vi "LabVIEW_Switch_State_Detection.vi"() -> ()   [LabVIEW 2020]
uses:
  <vilib>/Instr/_visa.llb/Select Event Type.ctl
  <vilib>/Instr/_visa.llb/VISA Configure Serial Port (Instr).vi
panel:
  in  "Stop":bool
  in  "Tab Control":T1(tab)
  out "Switch 1":bool
  out "Serial Read Buffer":string
  in  "VISA resource name":refnum<visa-resource-name>="COM17"
  in  "baud rate (9600)":u32=9600
  out "Reading Rate (ms)":u32
  out "Switch 2":bool
  # "Switch State Detection with Arduino and LabVIEW"
  # "Auther: Suparat Yeamkuan\nOverview: Demonstrates the use of Arduino detect the state of a switch to LabVIEW.\nRequirements: Arduino UNO, Button Switch Modules, and  NI-VISA Driver."
  # "Instructions:\n1. Wiring soil moisture sensor to Arduino board follow below:"
  # "Instructions:\n1. Connect USB cable from Arduino board to computer.\n2. Use Arduino IDE to upload the code to Arduino board."
  # "Instructions:\n1. Select the VISA resource name as a COM port that Arduino connect to computer, this can show the COM port device manager.\n2. Run the VI.\n3. If your Arduino is reading voltage from sensor, it should show a response in the \"Serial Read Buffer\" and Voltage of Soil Moisture Sensor Chart."
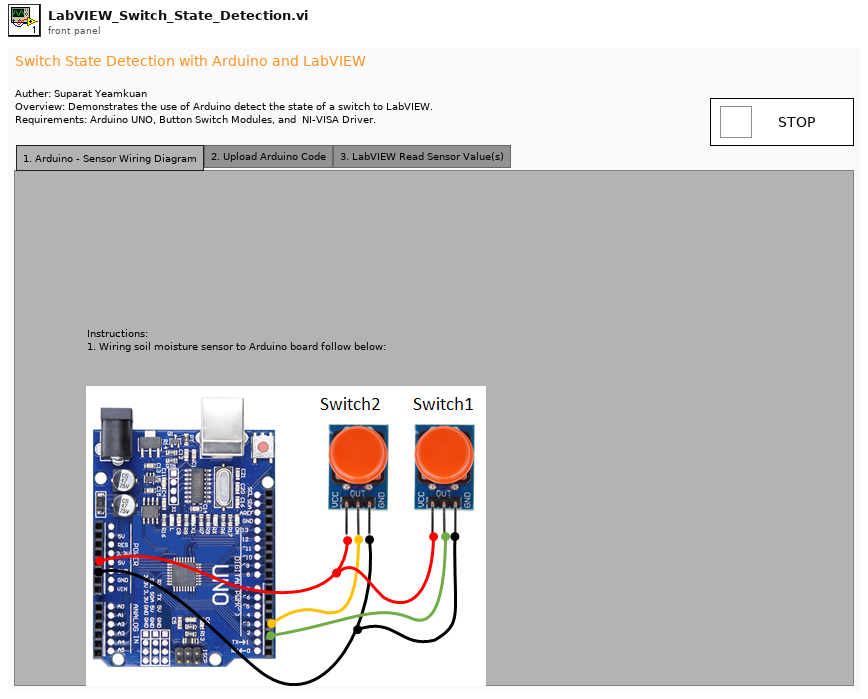
[diagram p1: front panel]
types:
  T1 = enum32{"1. Arduino - Sensor Wiring Diagram", "2. Upload Arduino Code", "3. LabVIEW Read Sensor Value(s)"}
  T2 = typedef "Select Event Type.ctl" = u32
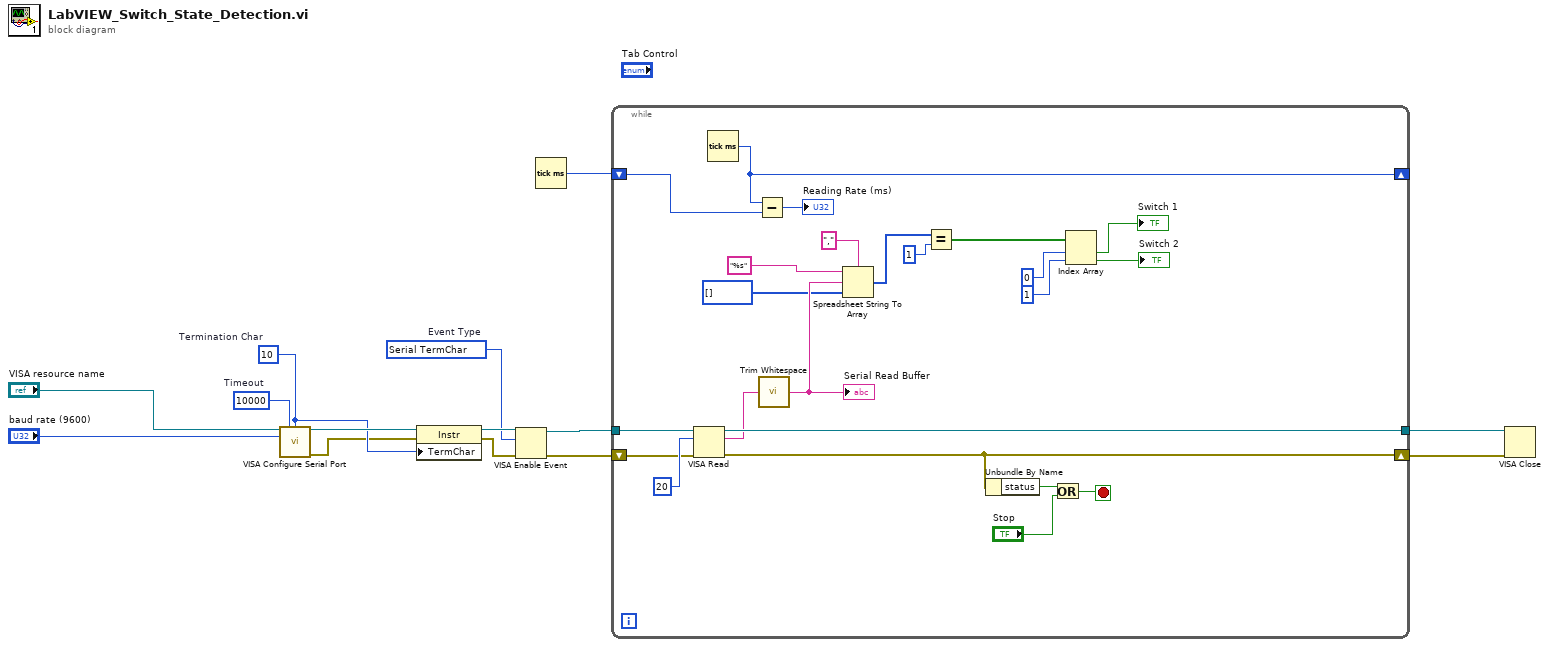
[diagram p0: block diagram]
diagram:
  w6 = T2 1073684516 items=["Service Request"=1073684491, "Trigger"=3221168138, "Clear"=1073684493, "VXI Signal"=1073684512, "VXI/VME Interrupt"=3221168161, "VXI/VME Sysfail"=1073684509, "VXI/VME Sysreset"=1073684510, "GPIB CIC"=1073684498, "GPIB Talk"=1073684499, "GPIB Listen"=1073684500, "PXI Interrupt"=1073684514, "Serial Break"=1073684515, "Serial TermChar"=1073684516, "Serial CTS"=1073684521, "Serial DSR"=1073684522, "Serial DCD"=1073684524, "Serial RI"=1073684526, "Serial Character"=1073684533, "USB Interrupt"=1073684535, "All Enabled"=1073709055]  # Event Type
  w10 = u8 10  # Termination Char
  w12 = u32 10000  # Timeout
  n1 = call-poly "VISA Configure Serial Port"("VISA resource name"="VISA resource name", "timeout (10sec)"=w12, "termination char\n(0xA = '\\n' = LF)"=w10, "baud rate (9600)"="baud rate (9600)") -> ("VISA resource name out"=w11:refnum<visa-resource-name>, "error out"=w9:errorcluster)  [unwired: 10 in]
  n2 = property class="Instr"(reference=w11, error in=w9, "TermChar"=w10) -> (reference out=w8:refnum<visa-resource-name>, error out=w7:errorcluster)
  n3 = VISA Enable Event(8:w7, 10:w6, 11:w8) -> (0:w5:errorcluster, 3:w4:refnum<visa-resource-name>)  [unwired: 1 in]
  n4 = Tick Count (ms)() -> (millisecond timer value=w1:u32)
  n5 = while {
    shift-right: [w36] -> w13
    shift-left: w5 -> [w31]
    tunnel: [w37] -> w14
    tunnel: w4 -> [w30]
    shift-right: [w28] -> _
    shift-left: w1 -> [w27]
    stop <- w34 stop-if-true
    n6 = VISA Read(VISA resource name=w30, byte count=u32 20, error in (no error)=w31) -> (VISA resource name out=w37:refnum<visa-resource-name>, read buffer=w29:string, error out=w36:errorcluster)  [unwired: 1 out]
    n7 = Tick Count (ms)() -> (millisecond timer value=w28:u32)
    n8 = Subtract(x=w28, y=w27) -> (x-y=→"Reading Rate (ms)":u32)
    n9 = call <vilib>:"Trim Whitespace.vi"("string"=w29) -> ("trimmed string"=w25:string)  [unwired: 1 in]
    "Serial Read Buffer" <- w25
    n10 = Spreadsheet String To Array(delimiter (Tab)=",", format string="%s", spreadsheet string=w25, array type (2D Dbl)=i32[] []) -> (array=w19:i32[])
    n11 = Equal?(x=w19, y=1) -> (x = y?=w15:bool[])
    n12 = Unbundle By Name(w36) -> ("status"=w35:bool)
    n13 = Or(x=w35, y="Stop") -> (x .or. y?=w34:bool)
    n14 = Index Array(array=w15, index #1=0 ("index"), index #2=1 ("index")) -> (element #1=→"Switch 1":bool, element #2=→"Switch 2":bool)
  }
  n15 = VISA Close(VISA resource name=w14, error in (no error)=w13) -> ()  [unwired: 1 out]
